vi "find volume extremes.vi"(9 "end of volume":bool, 10 "current location":T1) -> (0 "min loc":T1, 3 "max loc":T1)   [LabVIEW 2010]
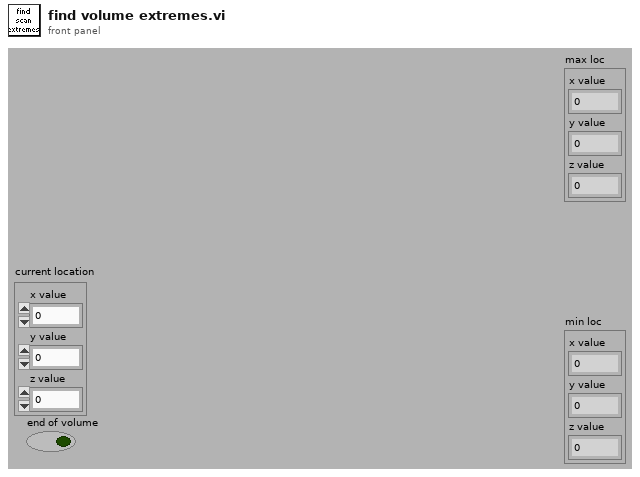
[diagram p1: front panel]
types:
  T1 = cluster{"x value":i16, "y value":i16, "z value":i16}
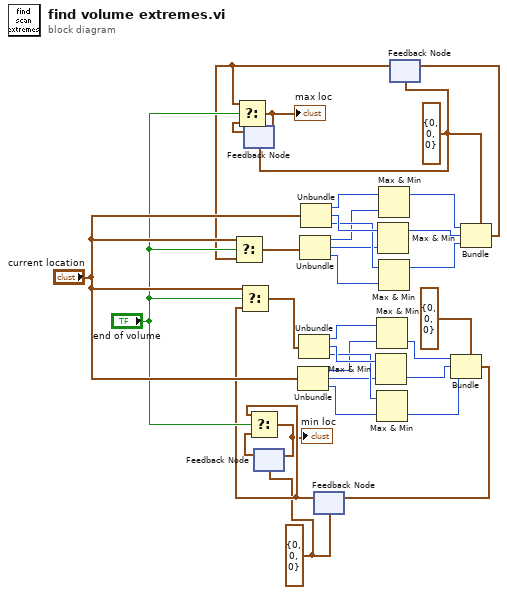
[diagram p0: block diagram]
diagram:
  w3 = T1 {"x value"=0, "y value"=0, "z value"=0} ("min loc in")
  w2 = T1 {"x value"=0, "y value"=0, "z value"=0} ("max loc out")
  n1 = feedback #1(w2) -> (w10:T1)
  n2 = feedback #2(w3) -> (w12:T1)
  n3 = Unbundle("current location") -> ("x value"=w20:i16, "y value"=w19:i16, "z value"=w18:i16)
  n4 = Unbundle("current location") -> ("x value"=w32:i16, "y value"=w31:i16, "z value"=w30:i16)
  n5 = feedback #3(w3) -> (w4:T1)
  n6 = Select(t="current location", s="end of volume", f=w4) -> (s? t:f=w17:T1)
  n7 = Select(t=w4, s="end of volume", f=w12) -> (s? t:f=w1:T1)
  "min loc" <- w1
  n8 = feedback-in #2(w1) -> ()
  n9 = Unbundle(w17) -> ("x value"=w23:i16, "y value"=w22:i16, "z value"=w21:i16)
  n10 = Max & Min(x=w22, y=w19) -> (min(x,y)=w14:i16)  [unwired: 1 out]
  n11 = Max & Min(x=w23, y=w20) -> (min(x,y)=w15:i16)  [unwired: 1 out]
  n12 = Max & Min(x=w21, y=w18) -> (min(x,y)=w13:i16)  [unwired: 1 out]
  n13 = feedback #4(w2) -> (w8:T1)
  n14 = Select(t="current location", s="end of volume", f=w8) -> (s? t:f=w33:T1)
  n15 = Select(t=w8, s="end of volume", f=w10) -> (s? t:f=w7:T1)
  "max loc" <- w7
  n16 = feedback-in #1(w7) -> ()
  n17 = Unbundle(w33) -> ("x value"=w29:i16, "y value"=w28:i16, "z value"=w27:i16)
  n18 = Max & Min(x=w31, y=w28) -> (max(x,y)=w25:i16)  [unwired: 1 out]
  n19 = Max & Min(x=w32, y=w29) -> (max(x,y)=w26:i16)  [unwired: 1 out]
  n20 = Max & Min(x=w30, y=w27) -> (max(x,y)=w24:i16)  [unwired: 1 out]
  n21 = Bundle(cluster=T1 {"x value"=0, "y value"=0, "z value"=0} ("min loc in"), "x value"=w15, "y value"=w14, "z value"=w13) -> (w5:T1)
  n22 = feedback-in #3(w5) -> ()
  n23 = Bundle(cluster=w2, "x value"=w26, "y value"=w25, "z value"=w24) -> (w9:T1)
  n24 = feedback-in #4(w9) -> ()
